vi "Test Reading and Writing Binary Config.vi"() -> ()   [LabVIEW 2021]
uses:
  Source/Bool/conc_SharedVar_Bool.lvclass
  C:/Program Files (x86)/National Instruments/LabVIEW 2021/vi.lib/TSA/Abstract Data Classes/Abs_Types/Type/Abs_Type.lvclass
  <vilib>/TSA/Abstract Data Classes/Abs_Types/Boolean/Abs_Boolean.lvclass
  <vilib>/TSA/Abstract Data Classes/Abs_Types/Type/Abs_Type.lvclass/Abs_Type.ctl
  <vilib>/TSA/Abstract Data Classes/Abs_Types/Type/Properties/Write Name.vi
  <vilib>/TSA/Abstract Data Classes/Abs_Types/Type/Abs_Type.lvclass
panel:
  in  "Bool":bool
  out "Boolean":bool
  in  "stop":bool
  out "Binary":string
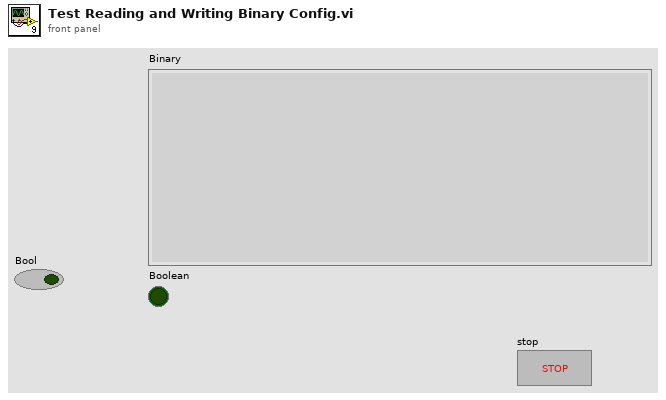
[diagram p1: front panel]
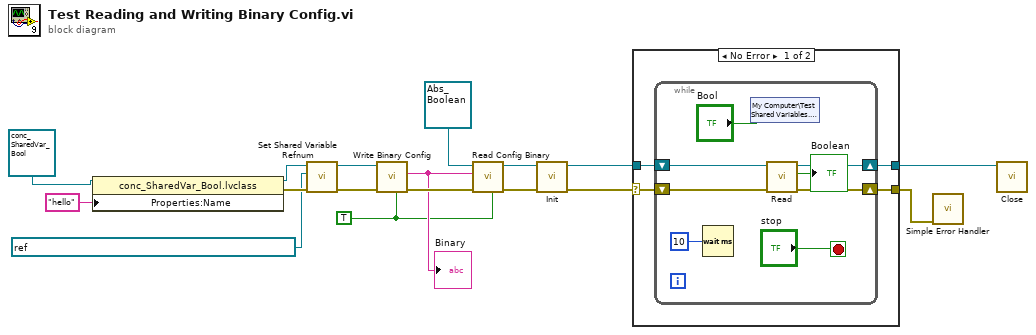
[diagram p0: block diagram]
diagram:
  w1 = TRUE ("Pretty Print?")
  n1 = property class="conc_SharedVar_Bool.lvclass"(reference=refnum<class "conc_SharedVar_Bool.lvclass"> refnum ("abs_SharedVar_Bool in"), "Properties:Name"="hello" ("Name")) -> (reference out=w6:refnum<class "conc_SharedVar_Bool.lvclass">, error out=w7:errorcluster)  [unwired: 1 in]
  n2 = call-dynamic "Set Shared Variable Refnum.vi"("error in (no error)"=w7, "shared variable refnum"=refnum<k21> "ni.var.psp://localhost/Test Shared Variables/Bool", "abs_SharedVar_Bool in"=w6) -> ("error out"=w3:errorcluster, "abs_SharedVar_Bool out"=w4:refnum<class "conc_SharedVar_Bool.lvclass">)  [unwired: 7 in]
  n3 = call-dynamic "Write Binary Config.vi"("Include Class Name"=w1, "error in (no error)"=w3, "abs_SharedVar_Bool in"=w4) -> ("error out"=w11:errorcluster, "Binary"=w8:string)  [unwired: 6 in, 1 out]
  "Binary" <- w8
  n4 = call <vilib>:"Read Config Binary.vi"("Class Name is Included"=w1, "error in (no error)"=w11, "Binary"=w8, "Abs_Type in"=refnum<class "Abs_Boolean.lvclass"> refnum ("Abs_Boolean.lvclass")) -> ("error out"=w12:errorcluster, "Abs_Type out"=w9:refnum<class "Abs_Boolean.lvclass">)  [unwired: 5 in, 1 out]
  n5 = call-dynamic "Init.vi"("error in (no error)"=w12, "Data in"=w9) -> ("error out"=w14:errorcluster, "Data out"=w15:refnum<class "Abs_Boolean.lvclass">)  [unwired: 8 in]
  n6 = case shown="No Error" w14 {
    selector: w14 -> [w20 w30]
    tunnel: w15 -> [w21 w31]
    tunnel: [w19 w31] -> w13
    tunnel: [w18 w30] -> w2
    frame No Error {
      n7 = while {
        shift-right: [w27] -> w19
        shift-left: w21 -> [w29]
        shift-right: [w26] -> w18
        shift-left: w20 -> [w28]
        stop <- "stop" stop-if-true
        n8 = Wait (ms)(milliseconds to wait=u32 10) -> ()  [unwired: 1 out]
        n9 = shared-variable "My Computer\\Test Shared Variables.lvlib\\Bool"("Bool") -> ()  [unwired: 1 in, 1 out]
        n10 = call-dynamic "Read.vi"("error in (no error)"=w28, "Boolean in"=w29) -> ("error out"=w26:errorcluster, "Boolean"=→"Boolean":bool, "Boolean out"=w27:refnum<class "Abs_Boolean.lvclass">)  [unwired: 7 in]
      }
    }
    frame Error {
    }
  }
  n11 = call <vilib>:"Simple Error Handler.vi"("error in (no error)"=w2) -> ()  [unwired: 4 in, 5 out]
  n12 = call-dynamic "Close.vi"("Data in"=w13) -> ()  [unwired: 9 in, 2 out]
